vi "Semantic_Voice_Array_Msg.vi"(8 "error in (no error)":errorcluster caption="错误输入（无错误）", 10 "值(信号)":T1, 11 "Guiding 输入":refnum<class "Voice.lvclass">) -> (0 "error out":errorcluster caption="错误输出", 3 "Process State out":refnum<class "State Actor.lvclass">)   [LabVIEW 2014, in "States.lvlib" / "Voice.lvclass"]
uses:
  Voice.lvclass
  <vilib>/NI/Actors/State Actor/State Actor/State Actor.lvclass
  ctl/Semantic_Voice_Array.ctl
  ctl/Point.ctl
  <vilib>/ActorFramework/Message Enqueuer/Message Enqueuer.lvclass/Message Enqueuer.ctl
  <vilib>/ActorFramework/Message Enqueuer/Enqueue.vi
  Global_var/Global_var.vi
  <vilib>/ActorFramework/Message Priority Queue/Priority Enqueue.vi
  Voice_lib/VoiceControl/Voice.lvclass
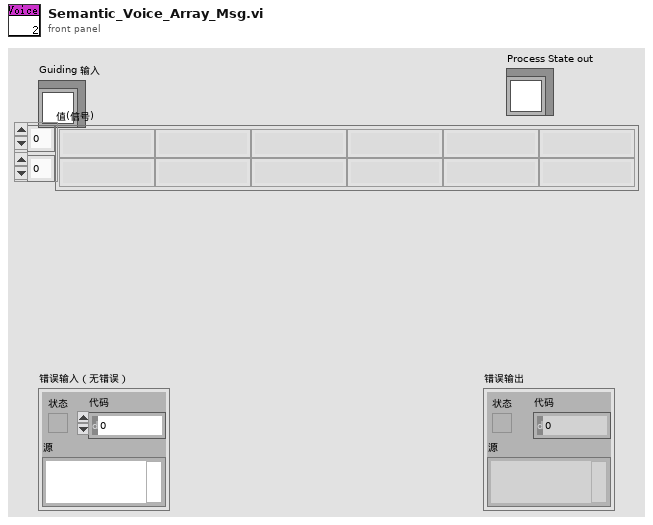
[diagram p1: front panel]
types:
  T1 = typedef "Semantic_Voice_Array.ctl" = string[][]
  T2 = cluster{"起点":string, "终点":string, "动作":string, "方向":string, "距离":string, "速度":string}
  T3 = typedef "Point.ctl" = cluster{"x":dbl, "y":dbl, "z":dbl}
  T4 = cluster{"now_pose_X":dbl, "now_pose_Y":dbl, "now_pose_Rot_deg":dbl}
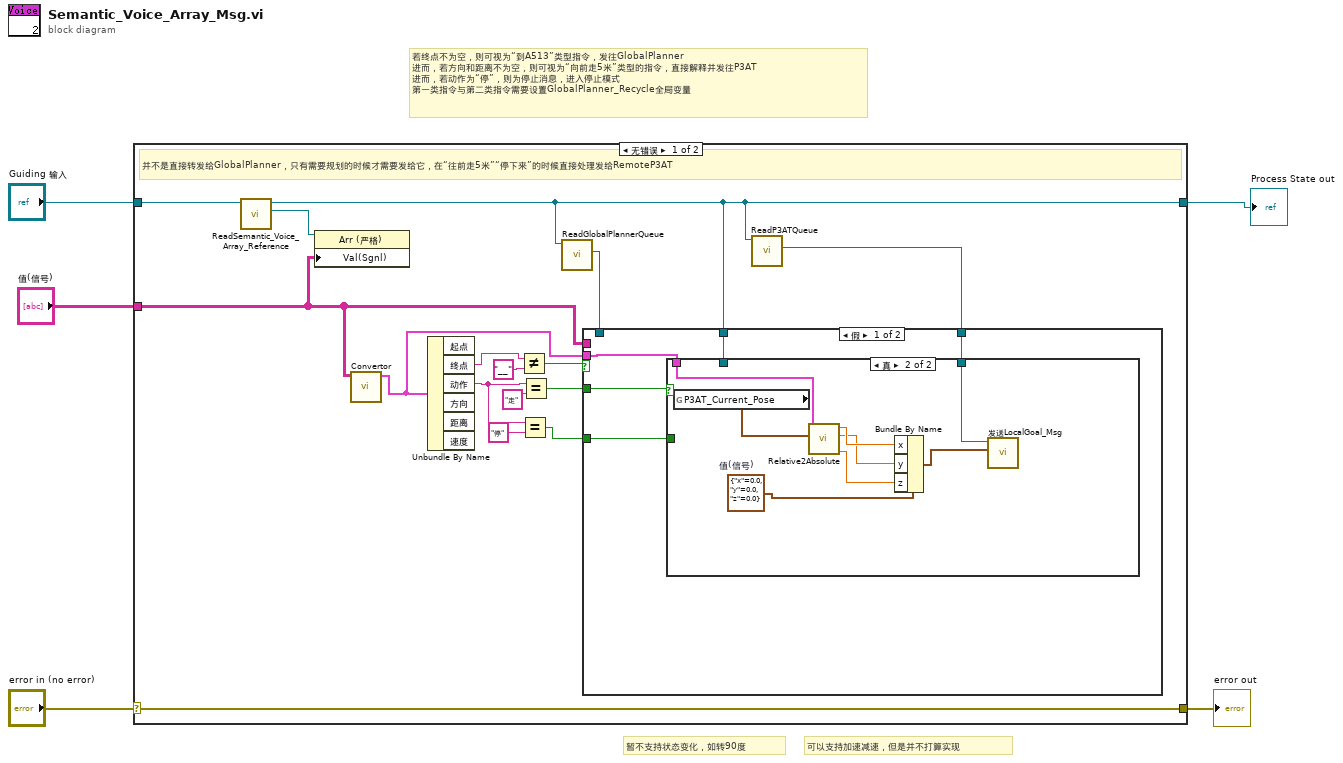
[diagram p0: block diagram]
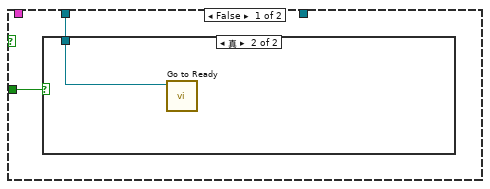
[diagram p2: hidden frame]
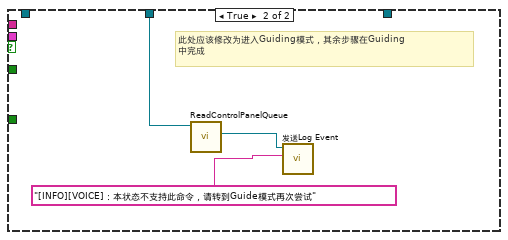
[diagram p4: hidden frame]
diagram:
  # "可以支持加速减速，但是并不打算实现"
  # "暂不支持状态变化，如转90度"
  # "若终点不为空，则可视为“到A513”类型指令，发往GlobalPlanner\n进而，若方向和距离不为空，则可视为“向前走5米”类型的指令，直接解释并发往P3AT\n进而，若动作为“停”，则为停止消息，进入停止模式\n第一类指令与第二类指令需要设置GlobalPlanner_Recycle全局变量"
  n1 = case shown="无错误" "error in (no error)" {
    selector: "error in (no error)" -> [w21 w42]
    tunnel: [w21 w42] -> w4
    tunnel: [w6 w41] -> w2
    tunnel: "Guiding 输入" -> [w20 w41]
    tunnel: "值(信号)" -> [w15 _]
    frame No Error {
      # "并不是直接转发给GlobalPlanner，只有需要规划的时候才需要发给它，在“往前走5米”“停下来”的时候直接处理发给RemoteP3AT"
      n2 = call-dynamic "ReadSemantic_Voice_Array_Reference.vi"("CoordinatorState输入"=w20) -> ("Semantic_Voice_Array_Reference"=w19:refnum<vi>, "CoordinatorState输出"=w6:refnum<class "Voice.lvclass">)  [unwired: 8 in, 1 out]
      n3 = property class="Arr (严格)"(reference=w19, "Val(Sgnl)"=w15) -> ()  [unwired: 1 in, 2 out]
      n4 = call "Convertor.vi"("机器人指令数组"=w15) -> ("机器人语音指令数据簇"=w11:T2)  [unwired: 10 in]
      n5 = Unbundle By Name(w11) -> ("终点"=w17:string, "动作"=w9:string)  [unwired: 4 out]
      n6 = Not Equal?(x=w17, y="__") -> (x != y?=w14:bool)
      n7 = Equal?(x=w9, y="停") -> (x = y?=w7:bool)
      n8 = Equal?(x=w9, y="走") -> (x = y?=w12:bool)
      n9 = call-dynamic "ReadGlobalPlannerQueue.vi"("CoordinatorState输入"=w6) -> ("操作者框架:消息待入队列"=w16:refnum<class "Message Enqueuer.lvclass">)  [unwired: 8 in, 2 out]
      n10 = call-dynamic "ReadP3ATQueue.vi"("CoordinatorState输入"=w6) -> ("操作者框架:消息待入队列"=w10:refnum<class "Message Enqueuer.lvclass">)  [unwired: 8 in, 2 out]
      n11 = case shown="假" w14 {
        tunnel: w16 -> [_ _]
        tunnel: w15 -> [_ _]
        tunnel: w12 -> [w26 _]
        tunnel: w11 -> [w25 _]
        tunnel: w10 -> [w24 _]
        tunnel: w7 -> [w23 _]
        tunnel: w6 -> [w22 w38]
        frame False {
          n12 = case shown="真" w26 {
            tunnel: w25 -> [_ w37]
            tunnel: w24 -> [_ w32]
            tunnel: w23 -> [w28 _]
            tunnel: w22 -> [w27 _]
            frame False {
              n13 = case shown="真" w28 {
                tunnel: w27 -> [_ w29]
                frame False {
                }
                frame True {
                  n14 = call-dynamic "Go to Ready.vi"("CommonState in"=w29) -> ()  [unwired: 9 in, 2 out]
                }
              }
            }
            frame True {
              w36 = T3 {"x"=0.0, "y"=0.0, "z"=0.0}  # 值(信号)
              n15 = global read "Global_var.vi" "P3AT_Current_Pose"() -> (w30:T4)
              n16 = call "Relative2Absolute.vi"("Ini_Pose"=w30, "机器人语音指令数据簇"=w37) -> ("Rot_deg"=w31:dbl, "y"=w34:dbl, "x"=w35:dbl)  [unwired: 7 in]
              n17 = Bundle By Name(cluster=w36, "x"=w35, "y"=w34, "z"=w31) -> (w33:T3)
              n18 = call "发送LocalGoal_Msg.vi"("值(信号)"=w33, "消息待入队列"=w32) -> ()  [unwired: 8 in, 2 out]
            }
          }
        }
        frame True {
          # "此处应该修改为进入Guiding模式，其余步骤在Guiding\n中完成"
          n19 = call-dynamic "ReadControlPanelQueue.vi"("CoordinatorState输入"=w38) -> ("操作者框架:消息待入队列"=w40:refnum<class "Message Enqueuer.lvclass">)  [unwired: 8 in, 2 out]
          n20 = call "发送Log Event.vi"("Event Text"="[INFO][VOICE]：本状态不支持此命令，请转到Guide模式再次尝试", "消息待入队列"=w40) -> ()  [unwired: 8 in, 2 out]
        }
      }
    }
    frame Error {
    }
  }
  "error out" <- w4
  "Process State out" <- w2
